vi "Post-Install Custom Action.vi"(10 "Variant":variant) -> (0 "error out":errorcluster)   [LabVIEW 2017]
uses:
  <vilib>/Utility/sysdir.llb/System Directory Type.ctl
  <vilib>/xml/Load XML File.vi
  <vilib>/xml/NI_XML.lvlib
  <resource>/objmgr/DOMUserDefRef.rc
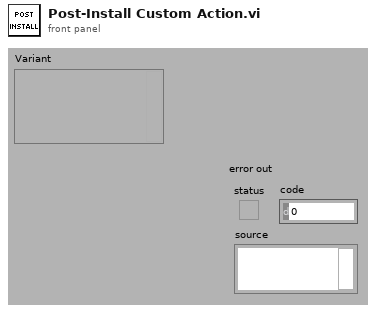
[diagram p1: front panel]
types:
  T1 = typedef "System Directory Type.ctl" = i32
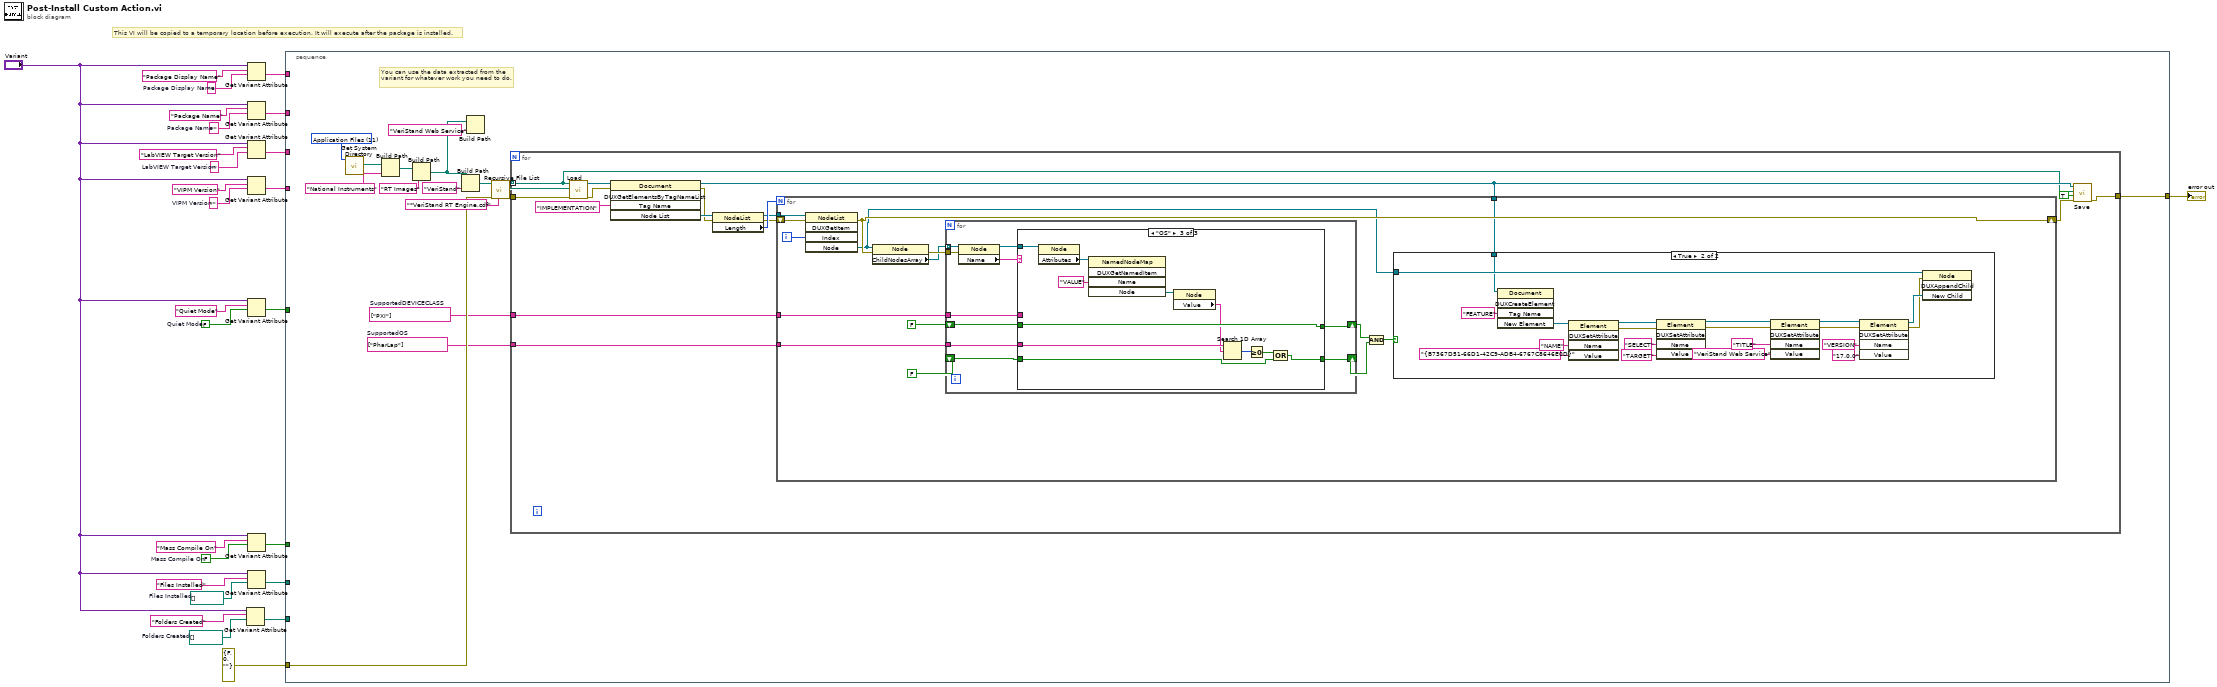
[diagram p0: block diagram]
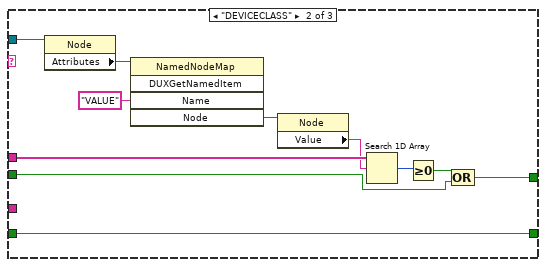
[diagram p4: hidden frame]
diagram:
  w3 = path[] []  # Folders Created
  w4 = path[] []  # Files Installed
  w10 = FALSE  # Mass Compile On
  w11 = ""  # Package Display Name
  w18 = FALSE  # Quiet Mode
  w21 = ""  # VIPM Version
  w23 = ""  # LabVIEW Target Version
  w25 = ""  # Package Name
  # "This VI will be copied to a temporary location before execution. It will execute after the package is installed."
  n1 = Get Variant Attribute(Variant="Variant", name="Folders Created", default value (empty Variant)=w3) -> (value=w8:path[])  [unwired: 1 in, 3 out]
  n2 = Get Variant Attribute(Variant="Variant", name="Package Display Name", default value (empty Variant)=w11) -> (value=w17:string)  [unwired: 1 in, 3 out]
  n3 = Get Variant Attribute(Variant="Variant", name="Package Name", default value (empty Variant)=w25) -> (value=w16:string)  [unwired: 1 in, 3 out]
  n4 = Get Variant Attribute(Variant="Variant", name="LabVIEW Target Version", default value (empty Variant)=w23) -> (value=w15:string)  [unwired: 1 in, 3 out]
  n5 = Get Variant Attribute(Variant="Variant", name="VIPM Version", default value (empty Variant)=w21) -> (value=w14:string)  [unwired: 1 in, 3 out]
  n6 = Get Variant Attribute(Variant="Variant", name="Quiet Mode", default value (empty Variant)=w18) -> (value=w13:bool)  [unwired: 1 in, 3 out]
  n7 = Get Variant Attribute(Variant="Variant", name="Mass Compile On", default value (empty Variant)=w10) -> (value=w12:bool)  [unwired: 1 in, 3 out]
  n8 = Get Variant Attribute(Variant="Variant", name="Files Installed", default value (empty Variant)=w4) -> (value=w7:path[])  [unwired: 1 in, 3 out]
  n9 = stacked-sequence {
    tunnel: w17 -> [_]
    tunnel: w16 -> [_]
    tunnel: w15 -> [_]
    tunnel: w14 -> [_]
    tunnel: w13 -> [_]
    tunnel: w12 -> [_]
    tunnel: w7 -> [_]
    tunnel: w8 -> [_]
    tunnel: errorcluster {"status"=FALSE, "code"=0, "source"=""} ("error out") -> [w35]
    tunnel: [w28] -> w1
    frame #0 {
      w31 = string[] ["PharLap"]  # SupportedOS
      w32 = string[] ["PXI"]  # SupportedDEVICECLASS
      w43 = T1 11 items=["User Home"=0, "User Desktop"=1, "User Documents"=2, "User Application Data"=3, "User Preferences"=4, "User Temporary"=5, "Public Documents"=6, "Public Application Data"=7, "Public Preferences"=8, "Public Cache"=13, "System Core Libraries"=9, "System Installed Libraries"=10, "Application Files"=11, "Boot Volume Root"=12] ("system directory type")
      # "You can use the data extracted from the variant for whatever work you need to do."
      n10 = call <vilib>:"Get System Directory.vi"("system directory type"=w43) -> ("system directory"=w42:path)  [unwired: 10 in]
      n11 = Build Path(base path=w42, name or relative path="National Instruments") -> (appended path=w40:path)
      n12 = Build Path(base path=w40, name or relative path="RT Images") -> (appended path=w30:path)
      n13 = Build Path(base path=w30, name or relative path="VeriStand") -> (appended path=w37:path)
      n14 = Build Path(base path=w30, name or relative path="VeriStand Web Service") -> ()  [unwired: 1 out]
      n15 = call <vilib>:"Recursive File List.vi"("pattern"="*VeriStand RT Engine.cdf", "error in (no error)"=w35, "Folder Path"=w37) -> ("error out"=w34:errorcluster, "All Files in Dir"=w33:path[])  [unwired: 4 in, 3 out]
      n16 = for {
        tunnel: w34 -> [w59]
        tunnel: w33 -> [w46] mode=indexing
        tunnel: w32 -> [w50]
        tunnel: w31 -> [w49]
        tunnel: [w44] -> w28
        n17 = call-poly <vilib>:"Load.vi"("path to XML document"=w46, "error in (no error)"=w59) -> ("DOM document out"=w58:refnum<k20>, "error out"=w56:errorcluster)  [unwired: 11 in, 1 out]
        n18 = invoke class="Document" method="DUXGetElementsByTagNameList"(reference=w58, error in=w56, "Tag Name"="IMPLEMENTATION") -> (reference out=w47:refnum<k20>, error out=w53:errorcluster, "Node List"=w55:refnum<k20>)  [unwired: 2 in, 2 out]
        n19 = property class="NodeList"(reference=w55, error in=w53) -> (reference out=w52:refnum<k20>, error out=w51:errorcluster, "Length"=w54:i32)
        n20 = for {
          N: w54 -> [_]
          tunnel: w52 -> [w74]
          shift-right: [w69] -> w48
          shift-left: w51 -> [w73]
          tunnel: w50 -> [w66]
          tunnel: w49 -> [w65]
          tunnel: w47 -> [w60]
          i -> [w72]
          n21 = invoke class="NodeList" method="DUXGetItem"(reference=w74, error in=w73, "Index"=w72) -> (error out=w69:errorcluster, "Node"=w61:refnum<k20>)  [unwired: 2 in, 3 out]
          n22 = property class="Node"(reference=w61, error in=w69) -> (error out=w71:errorcluster, "ChildNodesArray"=w70:refnum<k20>[])  [unwired: 1 out]
          n23 = for {
            tunnel: w71 -> [w104]
            tunnel: w70 -> [w103] mode=indexing
            shift-right: [w98] -> w64
            shift-left: FALSE -> [w101]
            shift-right: [w96] -> w63
            shift-left: FALSE -> [w97]
            tunnel: w66 -> [w100]
            tunnel: w65 -> [w95]
            n24 = property class="Node"(reference=w103, error in=w104) -> (reference out=w99:refnum<k20>, "Name"=w102:string)  [unwired: 1 out]
            n25 = case shown="\"OS\"" w102 {
              tunnel: w101 -> [w106 w109 w119]
              tunnel: w100 -> [_ w113 _]
              tunnel: w99 -> [_ w116 w127]
              tunnel: [w106 w108 w119] -> w98
              tunnel: w97 -> [w105 w107 w121]
              tunnel: [w105 w107 w120] -> w96
              tunnel: w95 -> [_ _ w122]
              frame Default {
              }
              frame "DEVICECLASS" {
                n26 = property class="Node"(reference=w116) -> ("Attributes"=w115:refnum<k20>)  [unwired: 1 in, 2 out]
                n27 = invoke class="NamedNodeMap" method="DUXGetNamedItem"(reference=w115, "Name"="VALUE") -> ("Node"=w112:refnum<k20>)  [unwired: 3 in, 4 out]
                n28 = property class="Node"(reference=w112) -> ("Value"=w111:string)  [unwired: 1 in, 2 out]
                n29 = Search 1D Array(1D array=w113, element=w111) -> (index of element=w117:i32)  [unwired: 1 in]
                n30 = Greater Or Equal To 0?(x=w117) -> (x >= 0?=w110:bool)
                n31 = Compound Arithmetic op=OR(w110, w109) -> (w108:bool)
              }
              frame "OS" {
                n32 = property class="Node"(reference=w127) -> ("Attributes"=w126:refnum<k20>)  [unwired: 1 in, 2 out]
                n33 = invoke class="NamedNodeMap" method="DUXGetNamedItem"(reference=w126, "Name"="VALUE") -> ("Node"=w124:refnum<k20>)  [unwired: 3 in, 4 out]
                n34 = property class="Node"(reference=w124) -> ("Value"=w118:string)  [unwired: 1 in, 2 out]
                n35 = Search 1D Array(1D array=w122, element=w118) -> (index of element=w128:i32)  [unwired: 1 in]
                n36 = Greater Or Equal To 0?(x=w128) -> (x >= 0?=w123:bool)
                n37 = Compound Arithmetic op=OR(w123, w121) -> (w120:bool)
              }
            }
          }
          n38 = Compound Arithmetic op=AND(w64, w63) -> (w62:bool)
          n39 = case shown="True" w62 {
            tunnel: w61 -> [_ w94]
            tunnel: w60 -> [_ w92]
            frame False {
            }
            frame True {
              n40 = invoke class="Document" method="DUXCreateElement"(reference=w92, "Tag Name"="FEATURE") -> ("New Element"=w91:refnum<k20>)  [unwired: 3 in, 4 out]
              n41 = invoke class="Element" method="DUXSetAttribute"(reference=w91, "Name"="NAME", "Value"="{B7367D51-66D1-42C9-ADB4-6767C8646E0D}") -> (reference out=w88:refnum<k20>, error out=w87:errorcluster)  [unwired: 2 in, 3 out]
              n42 = invoke class="Element" method="DUXSetAttribute"(reference=w88, error in=w87, "Name"="SELECT", "Value"="TARGET") -> (reference out=w84:refnum<k20>, error out=w83:errorcluster)  [unwired: 1 in, 3 out]
              n43 = invoke class="Element" method="DUXSetAttribute"(reference=w84, error in=w83, "Name"="TITLE", "Value"="VeriStand Web Service") -> (reference out=w80:refnum<k20>, error out=w79:errorcluster)  [unwired: 1 in, 3 out]
              n44 = invoke class="Element" method="DUXSetAttribute"(reference=w80, error in=w79, "Name"="VERSION", "Value"="17.0.0") -> (reference out=w76:refnum<k20>, error out=w75:errorcluster)  [unwired: 1 in, 3 out]
              n45 = invoke class="Node" method="DUXAppendChild"(reference=w94, error in=w75, "New Child"=w76) -> ()  [unwired: 1 in, 4 out]
            }
          }
        }
        n46 = call <vilib>:"Save.vi"("error in (no error)"=w48, "overwrite file (True)"=TRUE, "XML file path"=w46, "DOM document in"=w47) -> ("error out"=w44:errorcluster)  [unwired: 5 in, 2 out]
      }
    }
  }
  "error out" <- w1
